vi "醫用壓力襪的自動挑選系統.vi"() -> ()   [LabVIEW 2014]
panel:
  out "String 2":string
  in  "C":string
  in  "B":string
  in  "A":string
  out "Best Size for you":string
  in  "OK Button 5":bool
  in  "OK Button 4":bool
  in  "OK Button 3":bool
  in  "OK Button 2":bool
  in  "String":string
  in  "Ankle 2":string
  in  "Calf 2":string
  in  "Knee 2":string
  in  "Thigh 2":string
  in  "NUM":string
  in  "Ankle":string
  in  "Calf":string
  in  "Knee":string
  in  "Thigh":string
  in  "OK Button":bool
  # "(cm)"
  # "(cm)"
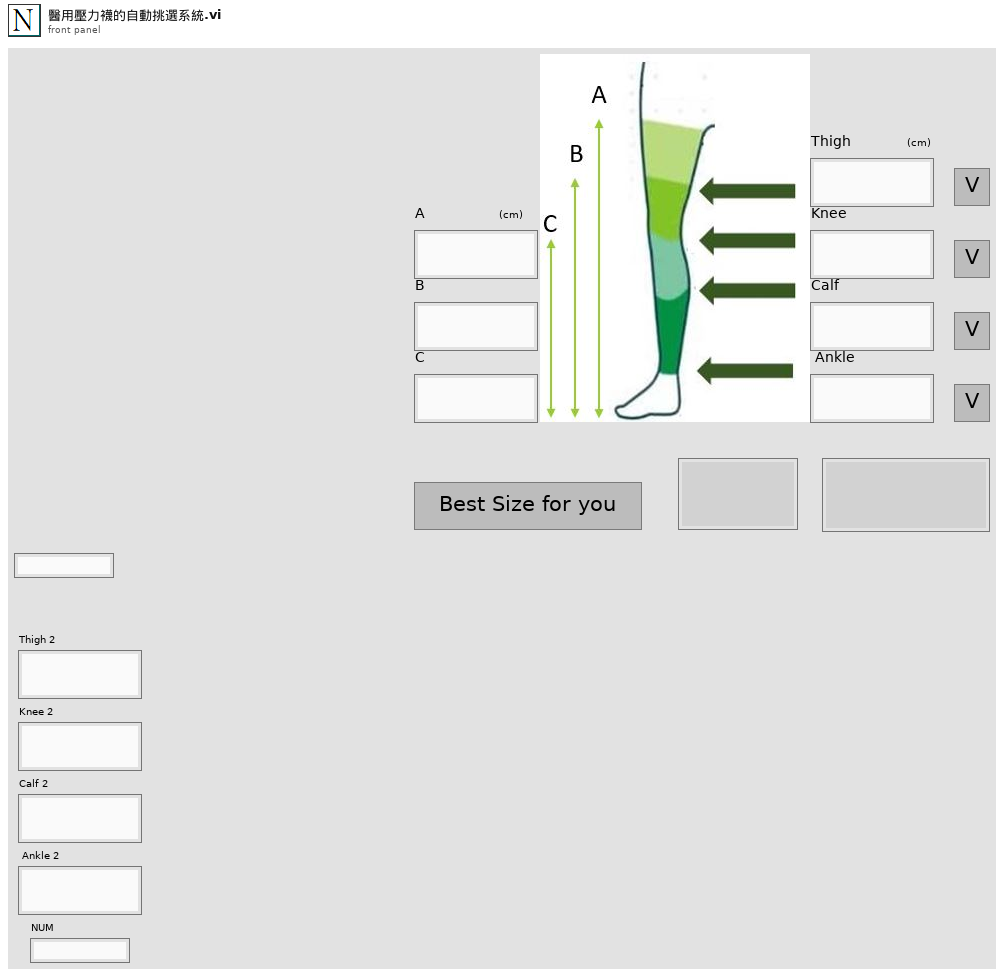
[diagram p1: front panel]
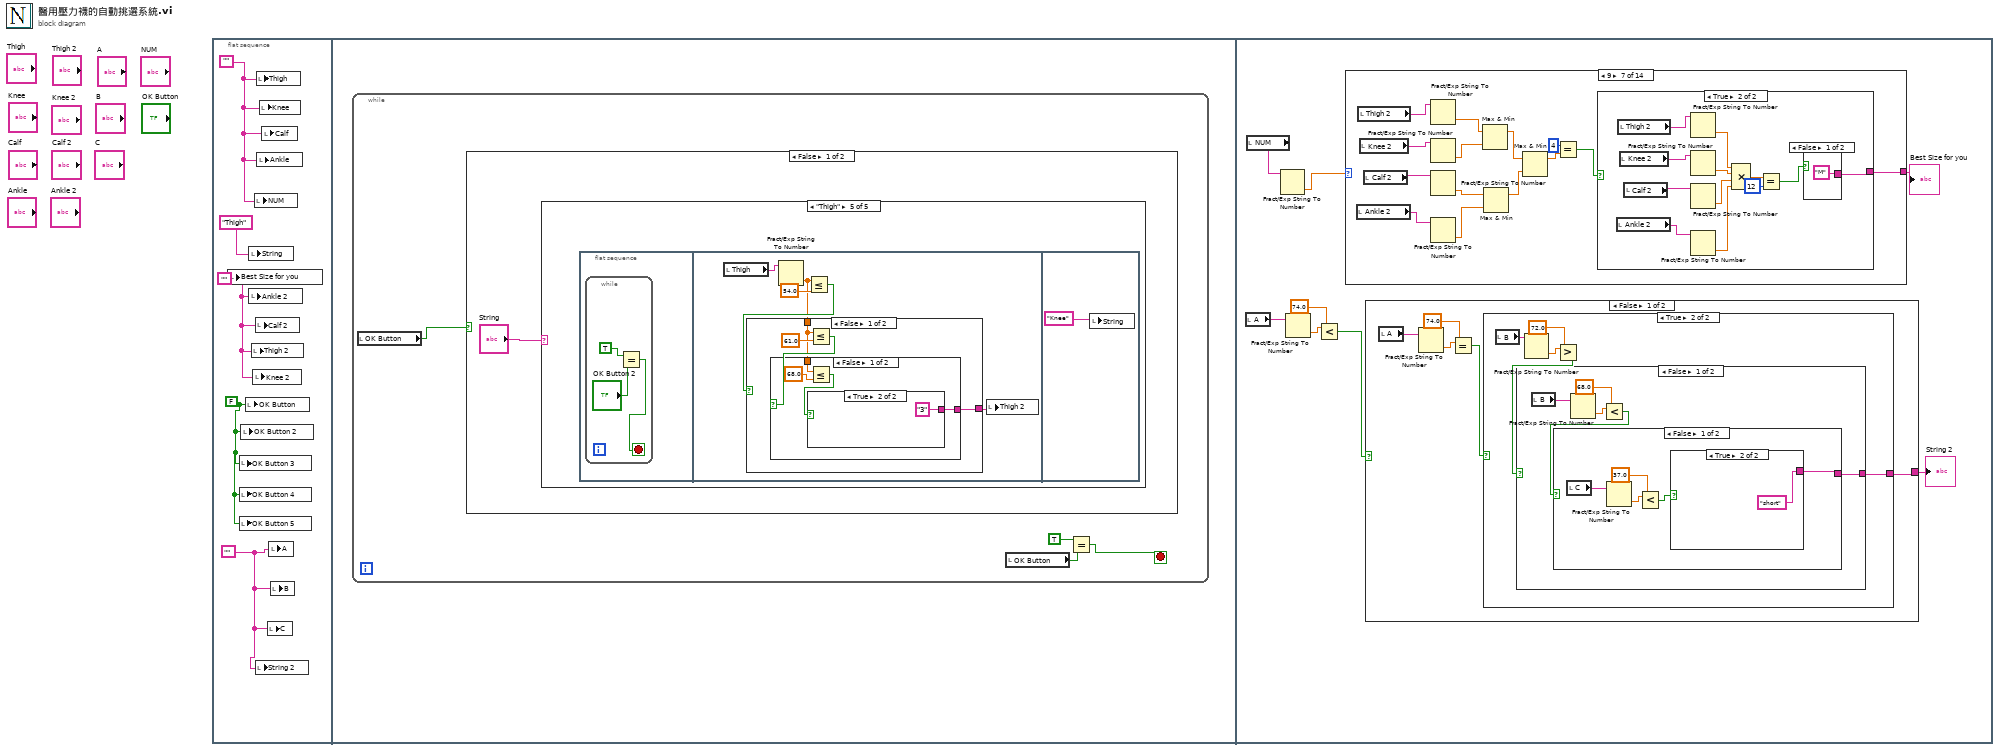
[diagram p0: block diagram]
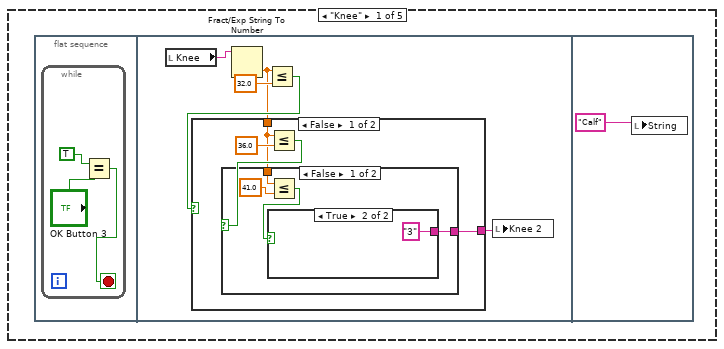
[diagram p2: hidden frame]
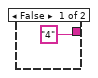
[diagram p3: hidden frame]
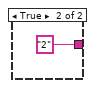
[diagram p4: hidden frame]
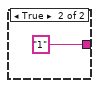
[diagram p5: hidden frame]
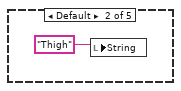
[diagram p6: hidden frame]
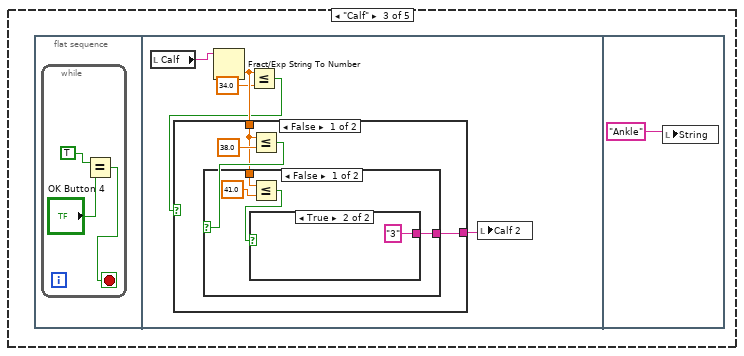
[diagram p7: hidden frame]
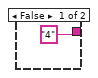
[diagram p8: hidden frame]
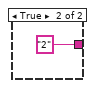
[diagram p9: hidden frame]
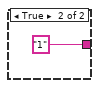
[diagram p10: hidden frame]
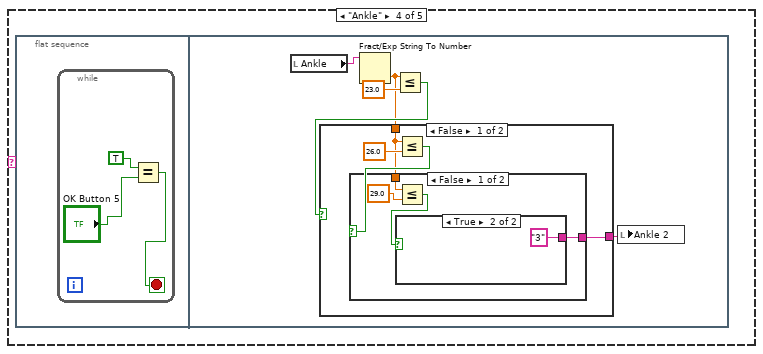
[diagram p11: hidden frame]
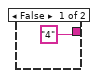
[diagram p12: hidden frame]
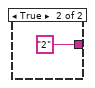
[diagram p13: hidden frame]
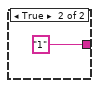
[diagram p14: hidden frame]
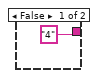
[diagram p15: hidden frame]
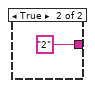
[diagram p16: hidden frame]
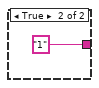
[diagram p17: hidden frame]
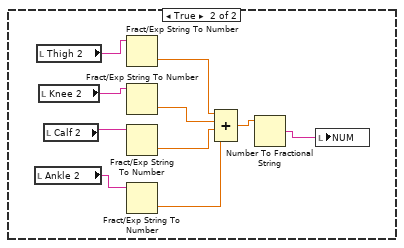
[diagram p18: hidden frame]
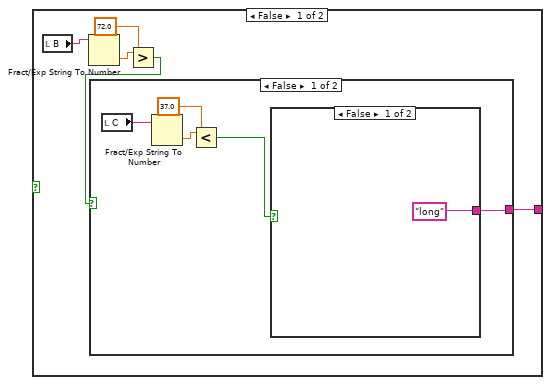
[diagram p19: hidden frame]
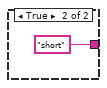
[diagram p20: hidden frame]
diagram:
  n1 = flat-sequence {
    frame #0 {
      w1 = ""
      w3 = FALSE
      w2 = ""
      w5 = ""
      n2 = local write "Best Size for you"(w2) -> ()
      n3 = local write "OK Button 3"(w3) -> ()
      n4 = local write "OK Button 4"(w3) -> ()
      n5 = local write "OK Button 5"(w3) -> ()
      n6 = local write "OK Button 2"(w3) -> ()
      n7 = local write "OK Button"(w3) -> ()
      n8 = local write "String"("Thigh") -> ()
      n9 = local write "Ankle 2"(w2) -> ()
      n10 = local write "Thigh 2"(w2) -> ()
      n11 = local write "Knee 2"(w2) -> ()
      n12 = local write "NUM"(w5) -> ()
      n13 = local write "Calf 2"(w2) -> ()
      n14 = local write "String 2"(w1) -> ()
      n15 = local write "Thigh"(w5) -> ()
      n16 = local write "Ankle"(w5) -> ()
      n17 = local write "Knee"(w5) -> ()
      n18 = local write "Calf"(w5) -> ()
      n19 = local write "C"(w1) -> ()
      n20 = local write "A"(w1) -> ()
      n21 = local write "B"(w1) -> ()
    }
    frame #1 {
      n22 = while {
        stop <- w6 stop-if-true
        n23 = local read "OK Button"() -> (w9:bool)
        n24 = case shown="False" w9 {
          frame False {
            n25 = case shown="\"Thigh\"" "String" {
              frame "Knee" {
                n26 = flat-sequence {
                  frame #0 {
                    n27 = while {
                      stop <- w11 stop-if-true
                      n28 = Equal?(x=TRUE, y="OK Button 3") -> (x = y?=w11:bool)
                    }
                  }
                  frame #1 {
                    n29 = local read "Knee"() -> (w18:string)
                    n30 = Fract/Exp String To Number(string=w18) -> (number=w14:dbl)  [unwired: 3 in, 1 out]
                    n31 = Less Or Equal?(x=w14, y=32.0) -> (x <= y?=w16:bool)
                    n32 = case shown="False" w16 {
                      tunnel: [w20 "1"] -> w15
                      tunnel: w14 -> [w19 _]
                      frame False {
                        n33 = Less Or Equal?(x=w19, y=36.0) -> (x <= y?=w21:bool)
                        n34 = case shown="False" w21 {
                          tunnel: [w23 "2"] -> w20
                          tunnel: w19 -> [w26 _]
                          frame False {
                            n35 = Less Or Equal?(x=w26, y=41.0) -> (x <= y?=w24:bool)
                            n36 = case shown="True" w24 {
                              tunnel: ["4" "3"] -> w23
                              frame False {
                              }
                              frame True {
                              }
                            }
                          }
                          frame True {
                          }
                        }
                      }
                      frame True {
                      }
                    }
                    n37 = local write "Knee 2"(w15) -> ()
                  }
                  frame #2 {
                    n38 = local write "String"("Calf") -> ()
                  }
                }
              }
              frame Default {
                n39 = local write "String"("Thigh") -> ()
              }
              frame "Calf" {
                n40 = flat-sequence {
                  frame #0 {
                    n41 = while {
                      stop <- w34 stop-if-true
                      n42 = Equal?(x=TRUE, y="OK Button 4") -> (x = y?=w34:bool)
                    }
                  }
                  frame #1 {
                    n43 = local read "Calf"() -> (w36:string)
                    n44 = Fract/Exp String To Number(string=w36) -> (number=w40:dbl)  [unwired: 3 in, 1 out]
                    n45 = Less Or Equal?(x=w40, y=34.0) -> (x <= y?=w38:bool)
                    n46 = case shown="False" w38 {
                      tunnel: [w42 "1"] -> w39
                      tunnel: w40 -> [w41 _]
                      frame False {
                        n47 = Less Or Equal?(x=w41, y=38.0) -> (x <= y?=w43:bool)
                        n48 = case shown="False" w43 {
                          tunnel: [w45 "2"] -> w42
                          tunnel: w41 -> [w48 _]
                          frame False {
                            n49 = Less Or Equal?(x=w48, y=41.0) -> (x <= y?=w46:bool)
                            n50 = case shown="True" w46 {
                              tunnel: ["4" "3"] -> w45
                              frame False {
                              }
                              frame True {
                              }
                            }
                          }
                          frame True {
                          }
                        }
                      }
                      frame True {
                      }
                    }
                    n51 = local write "Calf 2"(w39) -> ()
                  }
                  frame #2 {
                    n52 = local write "String"("Ankle") -> ()
                  }
                }
              }
              frame "Ankle" {
                n53 = flat-sequence {
                  frame #0 {
                    n54 = while {
                      stop <- w55 stop-if-true
                      n55 = Equal?(x=TRUE, y="OK Button 5") -> (x = y?=w55:bool)
                    }
                  }
                  frame #1 {
                    n56 = local read "Ankle"() -> (w61:string)
                    n57 = Fract/Exp String To Number(string=w61) -> (number=w57:dbl)  [unwired: 3 in, 1 out]
                    n58 = Less Or Equal?(x=w57, y=23.0) -> (x <= y?=w59:bool)
                    n59 = case shown="False" w59 {
                      tunnel: [w63 "1"] -> w58
                      tunnel: w57 -> [w62 _]
                      frame False {
                        n60 = Less Or Equal?(x=w62, y=26.0) -> (x <= y?=w64:bool)
                        n61 = case shown="False" w64 {
                          tunnel: [w66 "2"] -> w63
                          tunnel: w62 -> [w69 _]
                          frame False {
                            n62 = Less Or Equal?(x=w69, y=29.0) -> (x <= y?=w67:bool)
                            n63 = case shown="True" w67 {
                              tunnel: ["4" "3"] -> w66
                              frame False {
                              }
                              frame True {
                              }
                            }
                          }
                          frame True {
                          }
                        }
                      }
                      frame True {
                      }
                    }
                    n64 = local write "Ankle 2"(w58) -> ()
                  }
                }
              }
              frame "Thigh" {
                n65 = flat-sequence {
                  frame #0 {
                    n66 = while {
                      stop <- w75 stop-if-true
                      n67 = Equal?(x=TRUE, y="OK Button 2") -> (x = y?=w75:bool)
                    }
                  }
                  frame #1 {
                    n68 = local read "Thigh"() -> (w81:string)
                    n69 = Fract/Exp String To Number(string=w81) -> (number=w77:dbl)  [unwired: 3 in, 1 out]
                    n70 = Less Or Equal?(x=w77, y=54.0) -> (x <= y?=w79:bool)
                    n71 = case shown="False" w79 {
                      tunnel: [w83 "1"] -> w78
                      tunnel: w77 -> [w82 _]
                      frame False {
                        n72 = Less Or Equal?(x=w82, y=61.0) -> (x <= y?=w84:bool)
                        n73 = case shown="False" w84 {
                          tunnel: [w86 "2"] -> w83
                          tunnel: w82 -> [w89 _]
                          frame False {
                            n74 = Less Or Equal?(x=w89, y=68.0) -> (x <= y?=w87:bool)
                            n75 = case shown="True" w87 {
                              tunnel: ["4" "3"] -> w86
                              frame False {
                              }
                              frame True {
                              }
                            }
                          }
                          frame True {
                          }
                        }
                      }
                      frame True {
                      }
                    }
                    n76 = local write "Thigh 2"(w78) -> ()
                  }
                  frame #2 {
                    n77 = local write "String"("Knee") -> ()
                  }
                }
              }
            }
          }
          frame True {
            n78 = local read "Ankle 2"() -> (w104:string)
            n79 = local read "Thigh 2"() -> (w101:string)
            n80 = local read "Knee 2"() -> (w102:string)
            n81 = local read "Calf 2"() -> (w103:string)
            n82 = Fract/Exp String To Number(string=w101) -> (number=w100:dbl)  [unwired: 3 in, 1 out]
            n83 = Fract/Exp String To Number(string=w102) -> (number=w99:dbl)  [unwired: 3 in, 1 out]
            n84 = Fract/Exp String To Number(string=w103) -> (number=w98:dbl)  [unwired: 3 in, 1 out]
            n85 = Fract/Exp String To Number(string=w104) -> (number=w97:dbl)  [unwired: 3 in, 1 out]
            n86 = Compound Arithmetic op=ADD(w100, w99, w98, w97) -> (w96:dbl)
            n87 = Number To Fractional String(number=w96) -> (F-format string=w95:string)  [unwired: 3 in]
            n88 = local write "NUM"(w95) -> ()
          }
        }
        n89 = local read "OK Button"() -> (w7:bool)
        n90 = Equal?(x=TRUE, y=w7) -> (x = y?=w6:bool)
      }
    }
    frame #2 {
      n91 = local read "A"() -> (w108:string)
      n92 = local read "NUM"() -> (w111:string)
      n93 = Fract/Exp String To Number(string=w111) -> (number=w110:dbl)  [unwired: 3 in, 1 out]
      n94 = Fract/Exp String To Number(string=w108) -> (number=w107:dbl)  [unwired: 3 in, 1 out]
      n95 = Less?(x=w107, y=74.0) -> (x < y?=w109:bool)
      n96 = case shown="9" w110 {
        tunnel: ["" "S" "S" w180 w192 w204 w233 w275 w291 w330 w358 "XL" "XL" "XL"] -> w112
        frame 0, Default {
        }
        frame 4 {
        }
        frame 5 {
        }
        frame 6 {
          n97 = local read "Ankle 2"() -> (w176:string)
          n98 = local read "Thigh 2"() -> (w179:string)
          n99 = local read "Knee 2"() -> (w178:string)
          n100 = local read "Calf 2"() -> (w177:string)
          n101 = Fract/Exp String To Number(string=w179) -> (number=w175:dbl)  [unwired: 3 in, 1 out]
          n102 = Fract/Exp String To Number(string=w178) -> (number=w174:dbl)  [unwired: 3 in, 1 out]
          n103 = Fract/Exp String To Number(string=w177) -> (number=w173:dbl)  [unwired: 3 in, 1 out]
          n104 = Fract/Exp String To Number(string=w176) -> (number=w172:dbl)  [unwired: 3 in, 1 out]
          n105 = Max & Min(x=w175, y=w174) -> (max(x,y)=w181:dbl)  [unwired: 1 out]
          n106 = Max & Min(x=w173, y=w172) -> (max(x,y)=w182:dbl)  [unwired: 1 out]
          n107 = Max & Min(x=w181, y=w182) -> (max(x,y)=w183:dbl)  [unwired: 1 out]
          n108 = Equal?(x=w183, y=2) -> (x = y?=w185:bool)
          n109 = case shown="False" w185 {
            tunnel: ["S" "M"] -> w180
            frame False {
            }
            frame True {
            }
          }
        }
        frame 7 {
          n110 = local read "Ankle 2"() -> (w198:string)
          n111 = local read "Thigh 2"() -> (w201:string)
          n112 = local read "Knee 2"() -> (w200:string)
          n113 = local read "Calf 2"() -> (w199:string)
          n114 = Fract/Exp String To Number(string=w201) -> (number=w191:dbl)  [unwired: 3 in, 1 out]
          n115 = Fract/Exp String To Number(string=w200) -> (number=w190:dbl)  [unwired: 3 in, 1 out]
          n116 = Fract/Exp String To Number(string=w199) -> (number=w189:dbl)  [unwired: 3 in, 1 out]
          n117 = Fract/Exp String To Number(string=w198) -> (number=w188:dbl)  [unwired: 3 in, 1 out]
          n118 = Max & Min(x=w191, y=w190) -> (max(x,y)=w197:dbl)  [unwired: 1 out]
          n119 = Max & Min(x=w189, y=w188) -> (max(x,y)=w196:dbl)  [unwired: 1 out]
          n120 = Max & Min(x=w197, y=w196) -> (max(x,y)=w195:dbl)  [unwired: 1 out]
          n121 = Greater Or Equal?(x=w195, y=3) -> (x >= y?=w193:bool)
          n122 = case shown="True" w193 {
            tunnel: ["M" "S"] -> w192
            frame False {
            }
            frame True {
            }
          }
        }
        frame 8 {
          n123 = local read "Ankle 2"() -> (w214:string)
          n124 = local read "Thigh 2"() -> (w217:string)
          n125 = local read "Knee 2"() -> (w216:string)
          n126 = local read "Calf 2"() -> (w215:string)
          n127 = Fract/Exp String To Number(string=w217) -> (number=w209:dbl)  [unwired: 3 in, 1 out]
          n128 = Fract/Exp String To Number(string=w216) -> (number=w208:dbl)  [unwired: 3 in, 1 out]
          n129 = Fract/Exp String To Number(string=w215) -> (number=w207:dbl)  [unwired: 3 in, 1 out]
          n130 = Fract/Exp String To Number(string=w214) -> (number=w206:dbl)  [unwired: 3 in, 1 out]
          n131 = Max & Min(x=w209, y=w208) -> (max(x,y)=w213:dbl)  [unwired: 1 out]
          n132 = Max & Min(x=w207, y=w206) -> (max(x,y)=w212:dbl)  [unwired: 1 out]
          n133 = Max & Min(x=w213, y=w212) -> (max(x,y)=w211:dbl)  [unwired: 1 out]
          n134 = Equal?(x=4, y=w211) -> (x = y?=w205:bool)
          n135 = case shown="False" w205 {
            tunnel: [w218 "S"] -> w204
            frame False {
              n136 = local read "Ankle 2"() -> (w229:string)
              n137 = local read "Thigh 2"() -> (w226:string)
              n138 = local read "Knee 2"() -> (w227:string)
              n139 = local read "Calf 2"() -> (w228:string)
              n140 = Fract/Exp String To Number(string=w226) -> (number=w222:dbl)  [unwired: 3 in, 1 out]
              n141 = Fract/Exp String To Number(string=w227) -> (number=w221:dbl)  [unwired: 3 in, 1 out]
              n142 = Fract/Exp String To Number(string=w228) -> (number=w220:dbl)  [unwired: 3 in, 1 out]
              n143 = Fract/Exp String To Number(string=w229) -> (number=w219:dbl)  [unwired: 3 in, 1 out]
              n144 = Compound Arithmetic op=MULTIPLY(w222, w221, w220, w219) -> (w225:dbl)
              n145 = Equal?(x=w225, y=9) -> (x = y?=w223:bool)
              n146 = case shown="False" w223 {
                tunnel: ["M" "L"] -> w218
                frame False {
                }
                frame True {
                }
              }
            }
            frame True {
            }
          }
        }
        frame 9 {
          n147 = local read "Ankle 2"() -> (w239:string)
          n148 = local read "Thigh 2"() -> (w242:string)
          n149 = local read "Knee 2"() -> (w241:string)
          n150 = local read "Calf 2"() -> (w240:string)
          n151 = Fract/Exp String To Number(string=w242) -> (number=w238:dbl)  [unwired: 3 in, 1 out]
          n152 = Fract/Exp String To Number(string=w241) -> (number=w237:dbl)  [unwired: 3 in, 1 out]
          n153 = Fract/Exp String To Number(string=w240) -> (number=w236:dbl)  [unwired: 3 in, 1 out]
          n154 = Fract/Exp String To Number(string=w239) -> (number=w235:dbl)  [unwired: 3 in, 1 out]
          n155 = Max & Min(x=w238, y=w237) -> (max(x,y)=w243:dbl)  [unwired: 1 out]
          n156 = Max & Min(x=w236, y=w235) -> (max(x,y)=w244:dbl)  [unwired: 1 out]
          n157 = Max & Min(x=w243, y=w244) -> (max(x,y)=w246:dbl)  [unwired: 1 out]
          n158 = Equal?(x=4, y=w246) -> (x = y?=w234:bool)
          n159 = case shown="True" w234 {
            tunnel: [w247 w269] -> w233
            frame False {
              n160 = local read "Ankle 2"() -> (w255:string)
              n161 = local read "Thigh 2"() -> (w258:string)
              n162 = local read "Knee 2"() -> (w257:string)
              n163 = local read "Calf 2"() -> (w256:string)
              n164 = Fract/Exp String To Number(string=w258) -> (number=w251:dbl)  [unwired: 3 in, 1 out]
              n165 = Fract/Exp String To Number(string=w257) -> (number=w250:dbl)  [unwired: 3 in, 1 out]
              n166 = Fract/Exp String To Number(string=w256) -> (number=w249:dbl)  [unwired: 3 in, 1 out]
              n167 = Fract/Exp String To Number(string=w255) -> (number=w248:dbl)  [unwired: 3 in, 1 out]
              n168 = Compound Arithmetic op=MULTIPLY(w251, w250, w249, w248) -> (w254:dbl)
              n169 = Equal?(x=w254, y=12) -> (x = y?=w252:bool)
              n170 = case shown="False" w252 {
                tunnel: ["M" "L"] -> w247
                frame False {
                }
                frame True {
                }
              }
            }
            frame True {
              n171 = local read "Ankle 2"() -> (w268:string)
              n172 = local read "Thigh 2"() -> (w265:string)
              n173 = local read "Knee 2"() -> (w266:string)
              n174 = local read "Calf 2"() -> (w267:string)
              n175 = Fract/Exp String To Number(string=w265) -> (number=w261:dbl)  [unwired: 3 in, 1 out]
              n176 = Fract/Exp String To Number(string=w266) -> (number=w262:dbl)  [unwired: 3 in, 1 out]
              n177 = Fract/Exp String To Number(string=w267) -> (number=w263:dbl)  [unwired: 3 in, 1 out]
              n178 = Fract/Exp String To Number(string=w268) -> (number=w264:dbl)  [unwired: 3 in, 1 out]
              n179 = Compound Arithmetic op=MULTIPLY(w261, w262, w263, w264) -> (w270:dbl)
              n180 = Equal?(x=w270, y=12) -> (x = y?=w272:bool)
              n181 = case shown="False" w272 {
                tunnel: ["M" "S"] -> w269
                frame False {
                }
                frame True {
                }
              }
            }
          }
        }
        frame 10 {
          n182 = local read "Ankle 2"() -> (w285:string)
          n183 = local read "Thigh 2"() -> (w288:string)
          n184 = local read "Knee 2"() -> (w287:string)
          n185 = local read "Calf 2"() -> (w286:string)
          n186 = Fract/Exp String To Number(string=w288) -> (number=w279:dbl)  [unwired: 3 in, 1 out]
          n187 = Fract/Exp String To Number(string=w287) -> (number=w278:dbl)  [unwired: 3 in, 1 out]
          n188 = Fract/Exp String To Number(string=w286) -> (number=w277:dbl)  [unwired: 3 in, 1 out]
          n189 = Fract/Exp String To Number(string=w285) -> (number=w276:dbl)  [unwired: 3 in, 1 out]
          n190 = Max & Min(x=w279, y=w278) -> (max(x,y)=w283:dbl)  [unwired: 1 out]
          n191 = Max & Min(x=w277, y=w276) -> (max(x,y)=w282:dbl)  [unwired: 1 out]
          n192 = Max & Min(x=w283, y=w282) -> (max(x,y)=w284:dbl)  [unwired: 1 out]
          n193 = Equal?(x=w284, y=4) -> (x = y?=w281:bool)
          n194 = case shown="True" w281 {
            tunnel: ["L" "XL"] -> w275
            frame False {
            }
            frame True {
            }
          }
        }
        frame 11 {
          n195 = local read "Ankle 2"() -> (w301:string)
          n196 = local read "Thigh 2"() -> (w304:string)
          n197 = local read "Knee 2"() -> (w303:string)
          n198 = local read "Calf 2"() -> (w302:string)
          n199 = Fract/Exp String To Number(string=w304) -> (number=w295:dbl)  [unwired: 3 in, 1 out]
          n200 = Fract/Exp String To Number(string=w303) -> (number=w294:dbl)  [unwired: 3 in, 1 out]
          n201 = Fract/Exp String To Number(string=w302) -> (number=w293:dbl)  [unwired: 3 in, 1 out]
          n202 = Fract/Exp String To Number(string=w301) -> (number=w292:dbl)  [unwired: 3 in, 1 out]
          n203 = Max & Min(x=w295, y=w294) -> (max(x,y)=w297:dbl)  [unwired: 1 out]
          n204 = Max & Min(x=w293, y=w292) -> (max(x,y)=w298:dbl)  [unwired: 1 out]
          n205 = Max & Min(x=w297, y=w298) -> (max(x,y)=w300:dbl)  [unwired: 1 out]
          n206 = Equal?(x=4, y=w300) -> (x = y?=w296:bool)
          n207 = case shown="False" w296 {
            tunnel: w295 -> [_ w309]
            tunnel: w294 -> [_ w308]
            tunnel: w293 -> [_ w307]
            tunnel: w292 -> [_ w306]
            tunnel: ["L" w310] -> w291
            frame False {
            }
            frame True {
              n208 = Compound Arithmetic op=MULTIPLY(w309, w308, w307, w306) -> (w312:dbl)
              n209 = Equal?(x=w312, y=32) -> (x = y?=w311:bool)
              n210 = case shown="False" w311 {
                tunnel: [w314 "XL"] -> w310
                tunnel: w309 -> [w319 _]
                tunnel: w308 -> [w318 _]
                tunnel: w307 -> [w317 _]
                tunnel: w306 -> [w316 _]
                frame False {
                  n211 = Compound Arithmetic op=MULTIPLY(w319, w318, w317, w316) -> (w321:dbl)
                  n212 = Equal?(x=w321, y=48) -> (x = y?=w315:bool)
                  n213 = case shown="False" w315 {
                    tunnel: ["L" "M"] -> w314
                    frame False {
                    }
                    frame True {
                    }
                  }
                }
                frame True {
                }
              }
            }
          }
        }
        frame 12 {
          n214 = local read "Ankle 2"() -> (w331:string)
          n215 = local read "Thigh 2"() -> (w334:string)
          n216 = local read "Knee 2"() -> (w333:string)
          n217 = local read "Calf 2"() -> (w332:string)
          n218 = Fract/Exp String To Number(string=w334) -> (number=w329:dbl)  [unwired: 3 in, 1 out]
          n219 = Fract/Exp String To Number(string=w333) -> (number=w328:dbl)  [unwired: 3 in, 1 out]
          n220 = Fract/Exp String To Number(string=w332) -> (number=w327:dbl)  [unwired: 3 in, 1 out]
          n221 = Fract/Exp String To Number(string=w331) -> (number=w326:dbl)  [unwired: 3 in, 1 out]
          n222 = Max & Min(x=w329, y=w328) -> (max(x,y)=w335:dbl)  [unwired: 1 out]
          n223 = Max & Min(x=w327, y=w326) -> (max(x,y)=w336:dbl)  [unwired: 1 out]
          n224 = Max & Min(x=w335, y=w336) -> (max(x,y)=w338:dbl)  [unwired: 1 out]
          n225 = Equal?(x=4, y=w338) -> (x = y?=w325:bool)
          n226 = case shown="True" w325 {
            tunnel: ["L" w344] -> w330
            tunnel: w329 -> [_ w343]
            tunnel: w328 -> [_ w342]
            tunnel: w327 -> [_ w341]
            tunnel: w326 -> [_ w340]
            frame False {
            }
            frame True {
              n227 = Compound Arithmetic op=MULTIPLY(w343, w342, w341, w340) -> (w347:dbl)
              n228 = Equal?(x=w347, y=72) -> (x = y?=w345:bool)
              n229 = case shown="True" w345 {
                tunnel: ["XL" "L"] -> w344
                frame False {
                }
                frame True {
                }
              }
            }
          }
        }
        frame 13 {
          n230 = local read "Ankle 2"() -> (w354:string)
          n231 = local read "Thigh 2"() -> (w357:string)
          n232 = local read "Knee 2"() -> (w356:string)
          n233 = local read "Calf 2"() -> (w355:string)
          n234 = Fract/Exp String To Number(string=w357) -> (number=w350:dbl)  [unwired: 3 in, 1 out]
          n235 = Fract/Exp String To Number(string=w356) -> (number=w351:dbl)  [unwired: 3 in, 1 out]
          n236 = Fract/Exp String To Number(string=w355) -> (number=w352:dbl)  [unwired: 3 in, 1 out]
          n237 = Fract/Exp String To Number(string=w354) -> (number=w353:dbl)  [unwired: 3 in, 1 out]
          n238 = Compound Arithmetic op=MULTIPLY(w350, w351, w352, w353) -> (w359:dbl)
          n239 = Equal?(x=w359, y=108) -> (x = y?=w361:bool)
          n240 = case shown="True" w361 {
            tunnel: ["XL" "L"] -> w358
            frame False {
            }
            frame True {
            }
          }
        }
        frame 14 {
        }
        frame 15 {
        }
        frame 16 {
        }
      }
      "Best Size for you" <- w112
      n241 = case shown="False" w109 {
        tunnel: [w113 w156] -> w105
        frame False {
          n242 = local read "A"() -> (w115:string)
          n243 = Fract/Exp String To Number(string=w115) -> (number=w116:dbl)  [unwired: 3 in, 1 out]
          n244 = Equal?(x=w116, y=74.0) -> (x = y?=w114:bool)
          n245 = case shown="True" w114 {
            tunnel: [w118 w131] -> w113
            frame False {
              n246 = local read "B"() -> (w120:string)
              n247 = Fract/Exp String To Number(string=w120) -> (number=w122:dbl)  [unwired: 3 in, 1 out]
              n248 = Greater?(x=w122, y=72.0) -> (0:w119:bool)
              n249 = case shown="False" w119 {
                tunnel: [w123 "long"] -> w118
                frame False {
                  n250 = local read "C"() -> (w125:string)
                  n251 = Fract/Exp String To Number(string=w125) -> (number=w126:dbl)  [unwired: 3 in, 1 out]
                  n252 = Less?(x=w126, y=37.0) -> (x < y?=w124:bool)
                  n253 = case shown="False" w124 {
                    tunnel: ["long" "short"] -> w123
                    frame False {
                    }
                    frame True {
                    }
                  }
                }
                frame True {
                }
              }
            }
            frame True {
              n254 = local read "B"() -> (w133:string)
              n255 = Fract/Exp String To Number(string=w133) -> (number=w135:dbl)  [unwired: 3 in, 1 out]
              n256 = Greater?(x=w135, y=72.0) -> (0:w132:bool)
              n257 = case shown="False" w132 {
                tunnel: [w136 "long"] -> w131
                frame False {
                  n258 = local read "B"() -> (w138:string)
                  n259 = Fract/Exp String To Number(string=w138) -> (number=w139:dbl)  [unwired: 3 in, 1 out]
                  n260 = Less?(x=w139, y=68.0) -> (x < y?=w137:bool)
                  n261 = case shown="False" w137 {
                    tunnel: [w142 w148] -> w136
                    frame False {
                      n262 = local read "C"() -> (w145:string)
                      n263 = Fract/Exp String To Number(string=w145) -> (number=w144:dbl)  [unwired: 3 in, 1 out]
                      n264 = Less?(x=w144, y=37.0) -> (x < y?=w141:bool)
                      n265 = case shown="True" w141 {
                        tunnel: ["long" "short"] -> w142
                        frame False {
                        }
                        frame True {
                        }
                      }
                    }
                    frame True {
                      n266 = local read "C"() -> (w152:string)
                      n267 = Fract/Exp String To Number(string=w152) -> (number=w151:dbl)  [unwired: 3 in, 1 out]
                      n268 = Less?(x=w151, y=37.0) -> (x < y?=w149:bool)
                      n269 = case shown="False" w149 {
                        tunnel: ["long" "short"] -> w148
                        frame False {
                        }
                        frame True {
                        }
                      }
                    }
                  }
                }
                frame True {
                }
              }
            }
          }
        }
        frame True {
          n270 = local read "B"() -> (w160:string)
          n271 = Fract/Exp String To Number(string=w160) -> (number=w159:dbl)  [unwired: 3 in, 1 out]
          n272 = Less?(x=w159, y=68.0) -> (x < y?=w157:bool)
          n273 = case shown="True" w157 {
            tunnel: [w161 "short"] -> w156
            frame False {
              n274 = local read "C"() -> (w163:string)
              n275 = Fract/Exp String To Number(string=w163) -> (number=w164:dbl)  [unwired: 3 in, 1 out]
              n276 = Less?(x=w164, y=37.0) -> (x < y?=w162:bool)
              n277 = case shown="False" w162 {
                tunnel: ["long" "short"] -> w161
                frame False {
                }
                frame True {
                }
              }
            }
            frame True {
            }
          }
        }
      }
      "String 2" <- w105
    }
  }
